vi "Automatic Teller Machine (ATM).vi"() -> ()   [LabVIEW 2015]
uses:
  Controls/State.ctl
  Controls/AccessModeFGV.ctl
panel:
  in  "Enter":bool
  in  "User Input":string
  in  "Right Buttons":T1
  out "Right Menu":T2
  in  "Left Buttons":T1
  out "Left Menu":T2
  in  "Card Simulator":bool
  out "ATM Messages":string
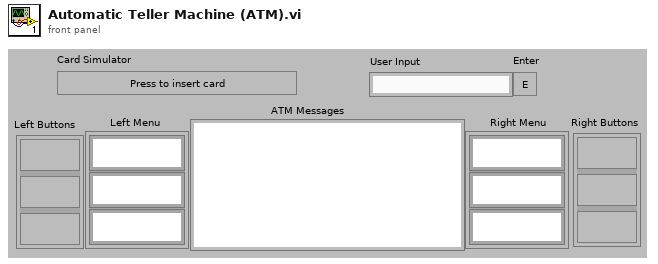
[diagram p1: front panel]
types:
  T1 = cluster{"Func Button":bool, "Func Button 2":bool, "Func Button 3":bool}
  T2 = cluster{"RFS String":string, "RFS String 2":string, "RFS String 3":string}
  T3 = typedef "AccessModeFGV.ctl" = enum16{"SearchUser", "Deposite", "Withdraw", "Fast Cash $50", "Balance Inquiry"}
  T4 = typedef "State.ctl" = enum16{"Init", "Start", "Work", "Stop"}
  T5 = enum8{"Enabled", "Disabled", "Disabled and Grayed Out"}
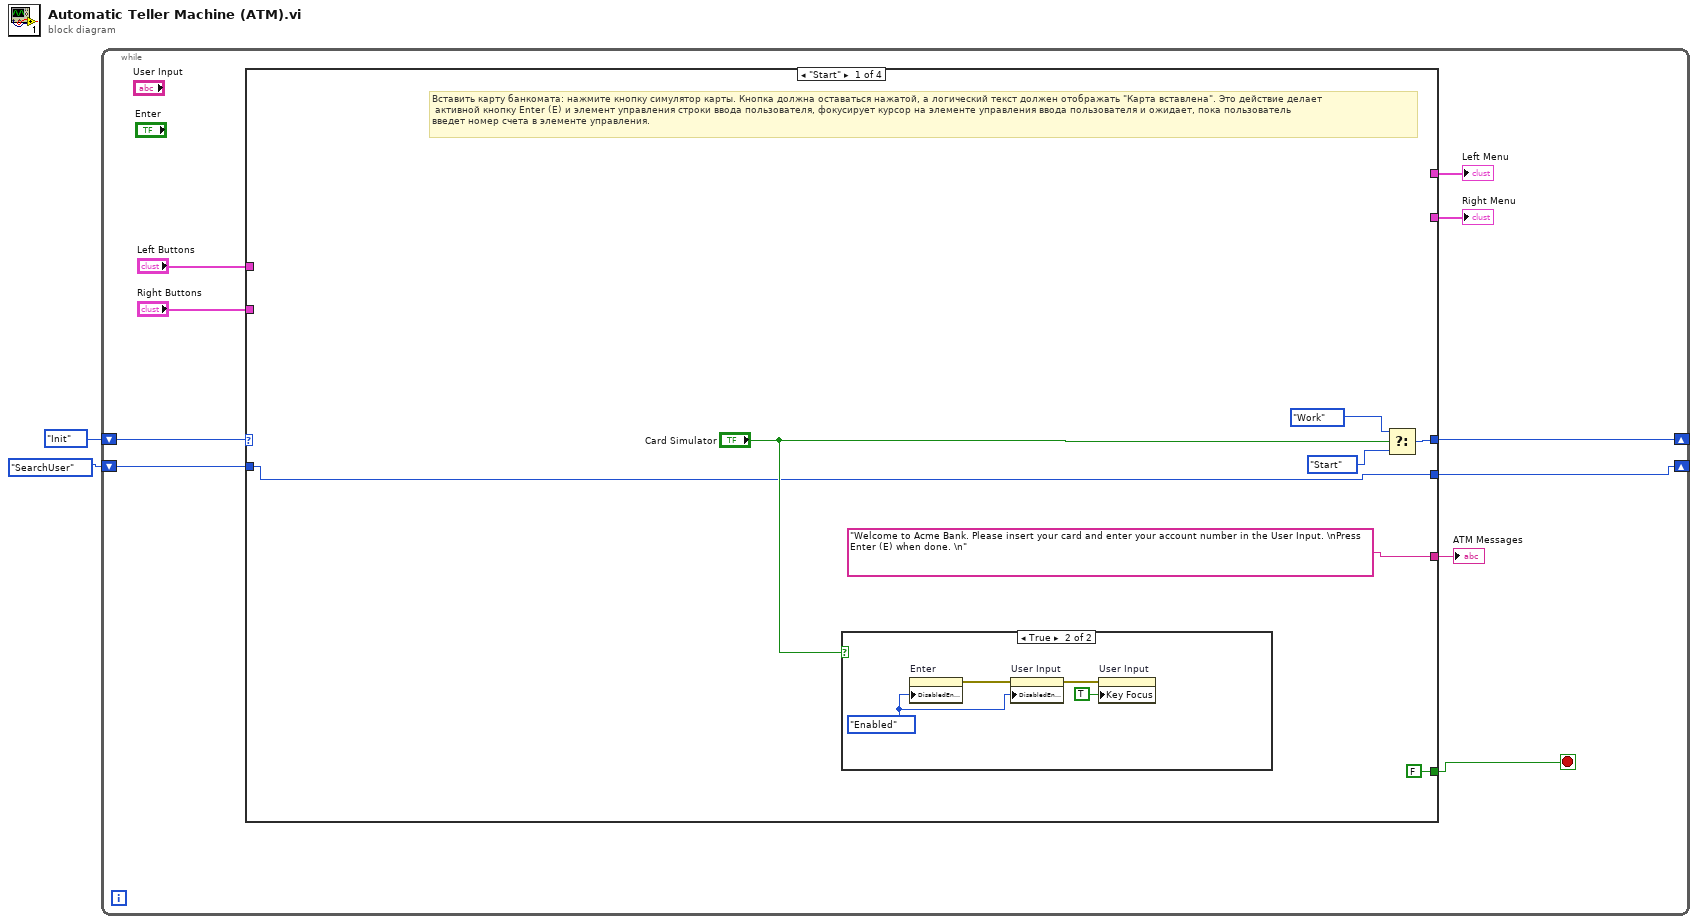
[diagram p0: block diagram]
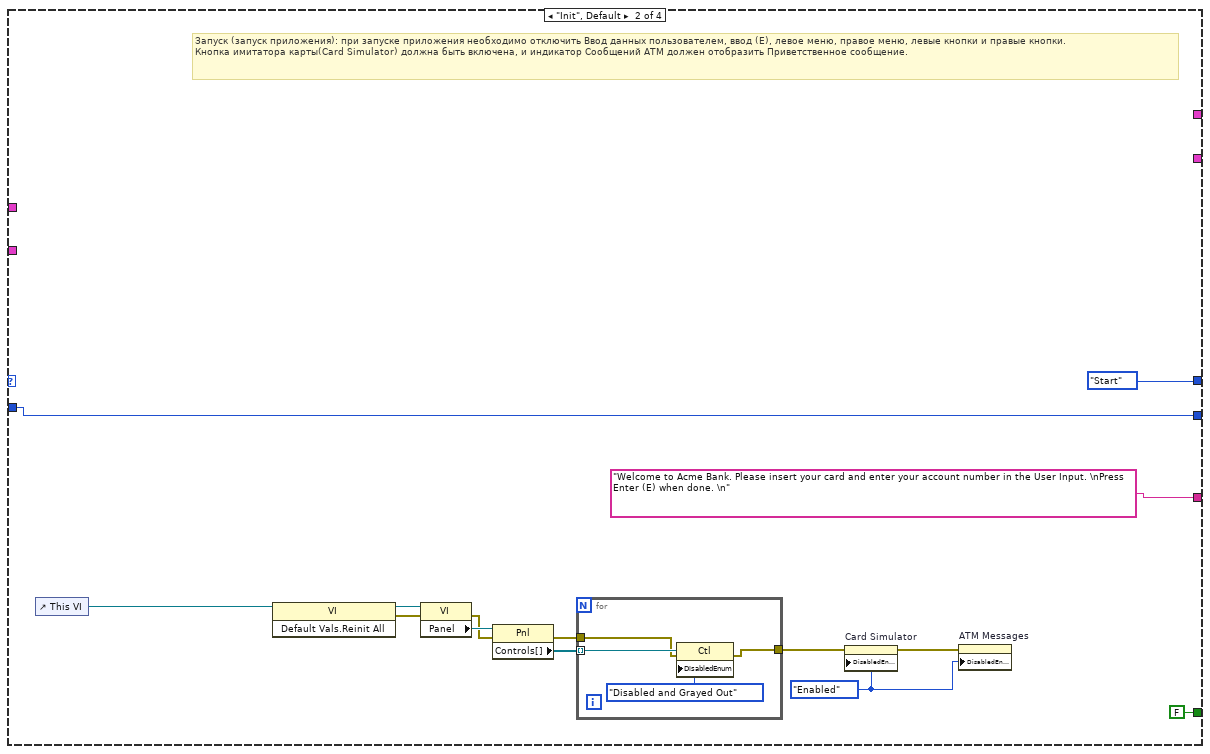
[diagram p3: hidden frame]
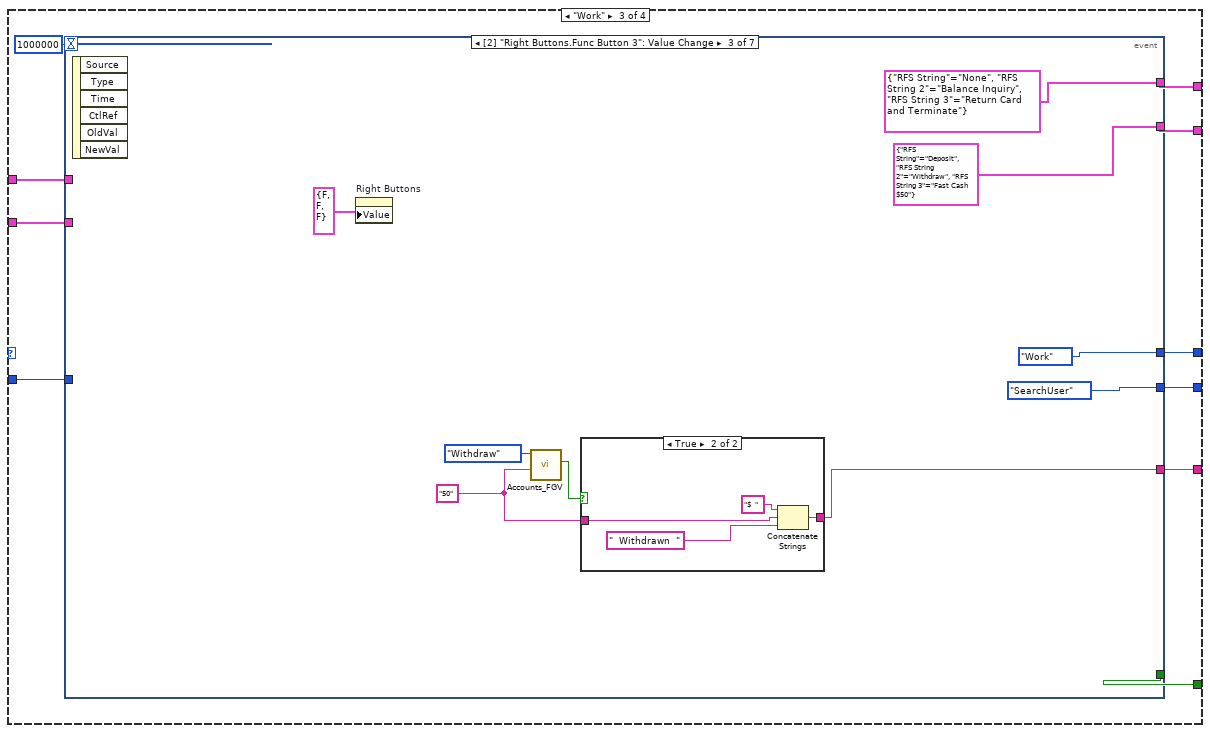
[diagram p4: hidden frame]
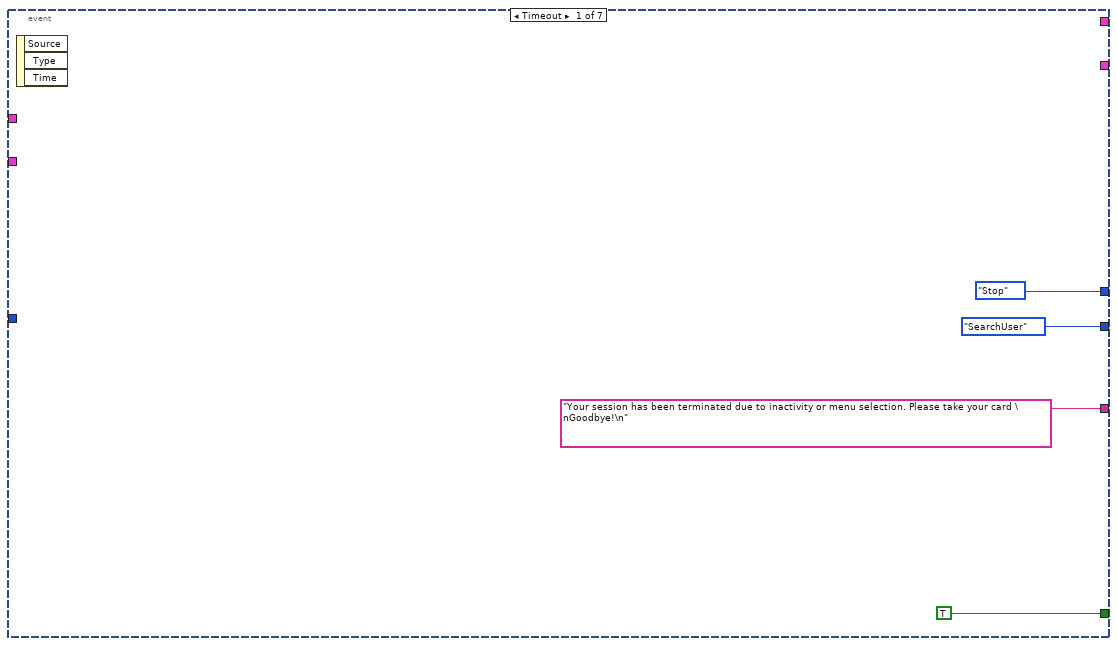
[diagram p5: hidden frame]
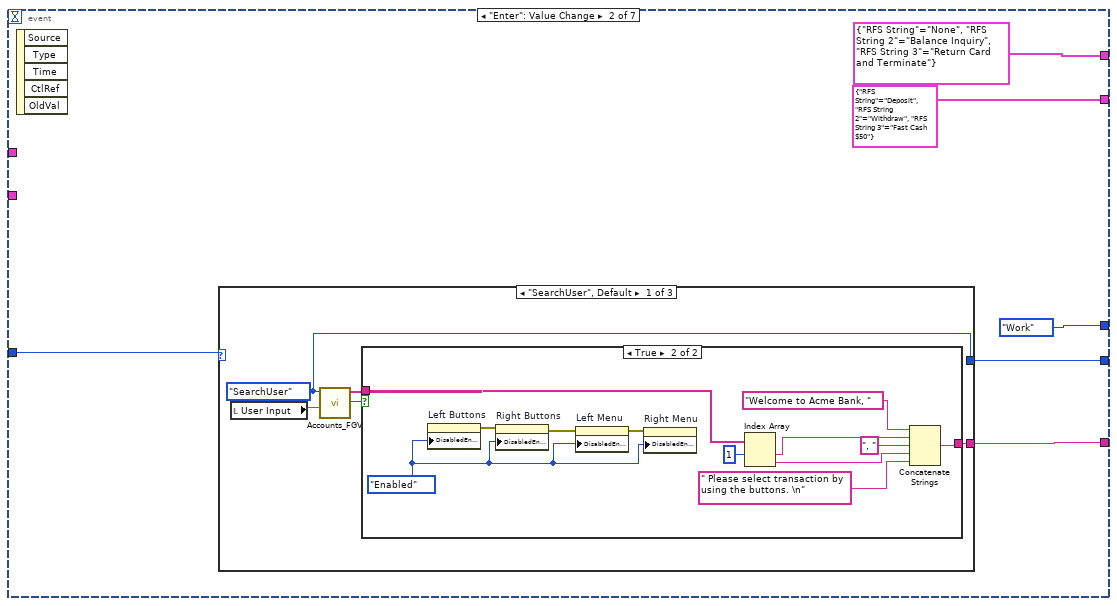
[diagram p6: hidden frame]
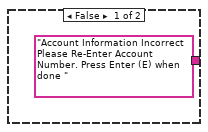
[diagram p7: hidden frame]
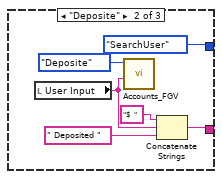
[diagram p8: hidden frame]
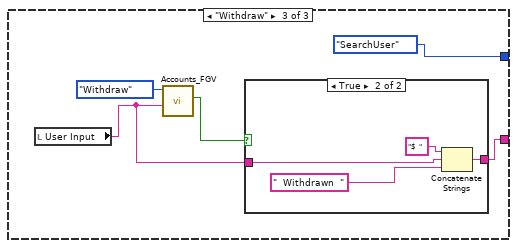
[diagram p9: hidden frame]
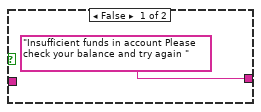
[diagram p10: hidden frame]
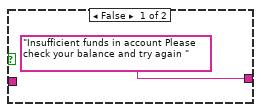
[diagram p11: hidden frame]
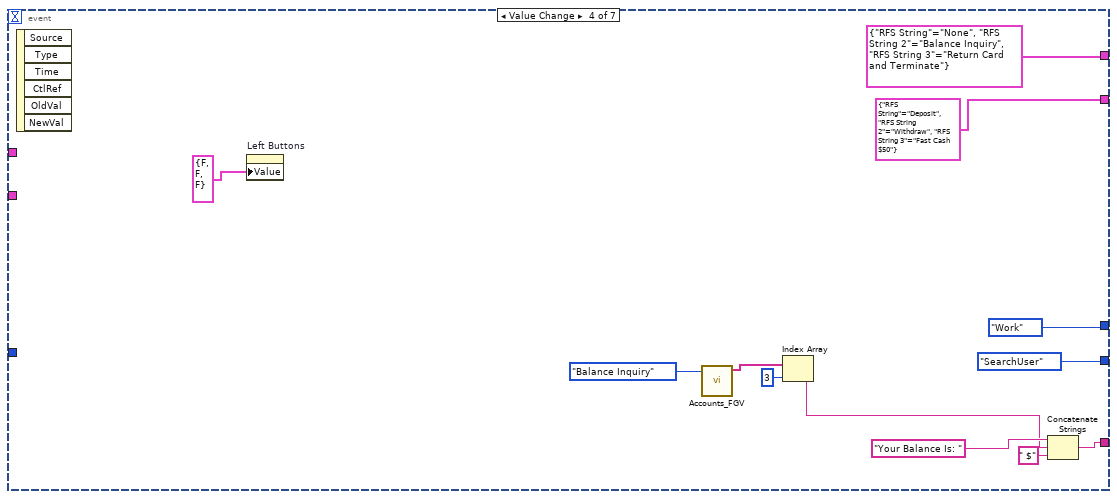
[diagram p12: hidden frame]
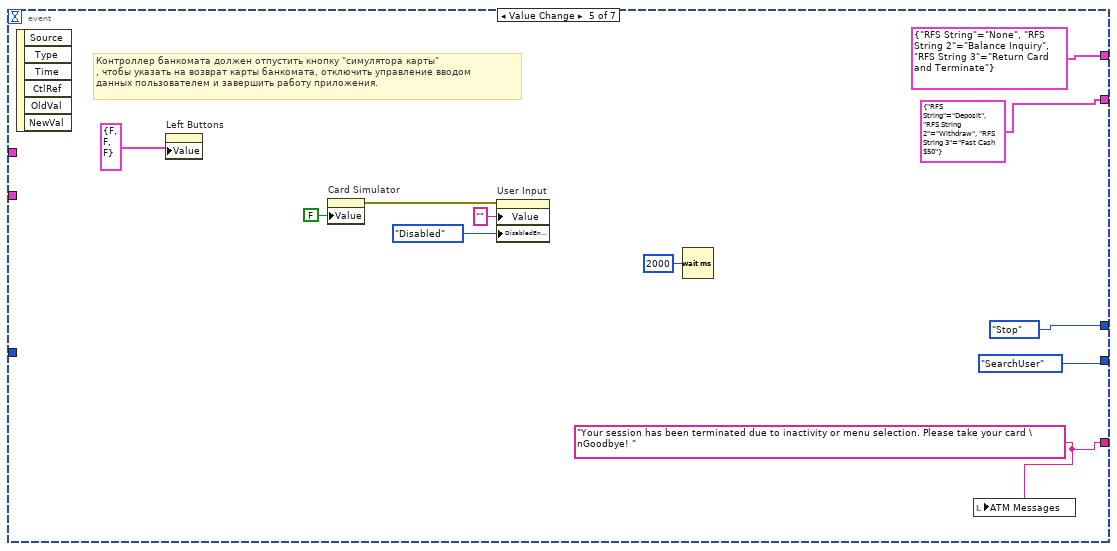
[diagram p13: hidden frame]
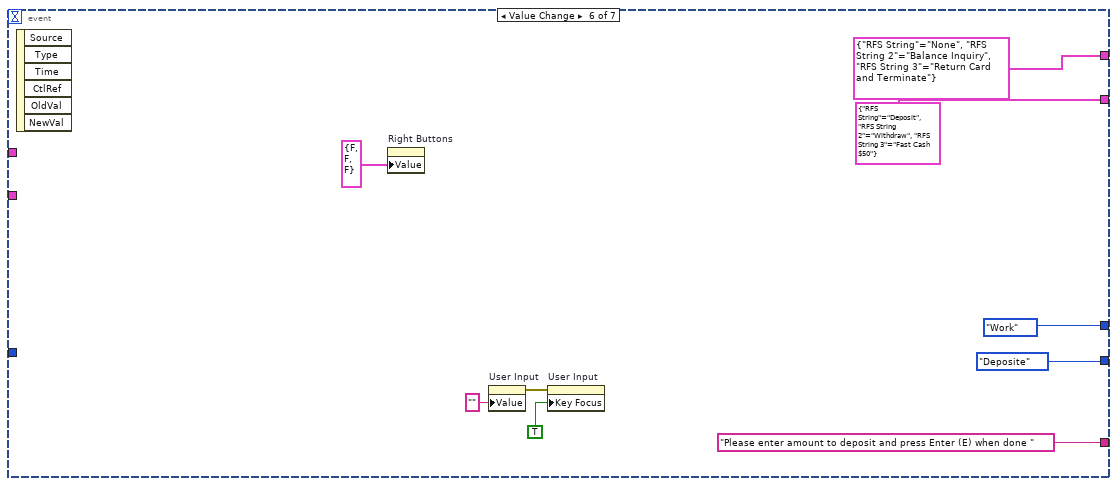
[diagram p14: hidden frame]
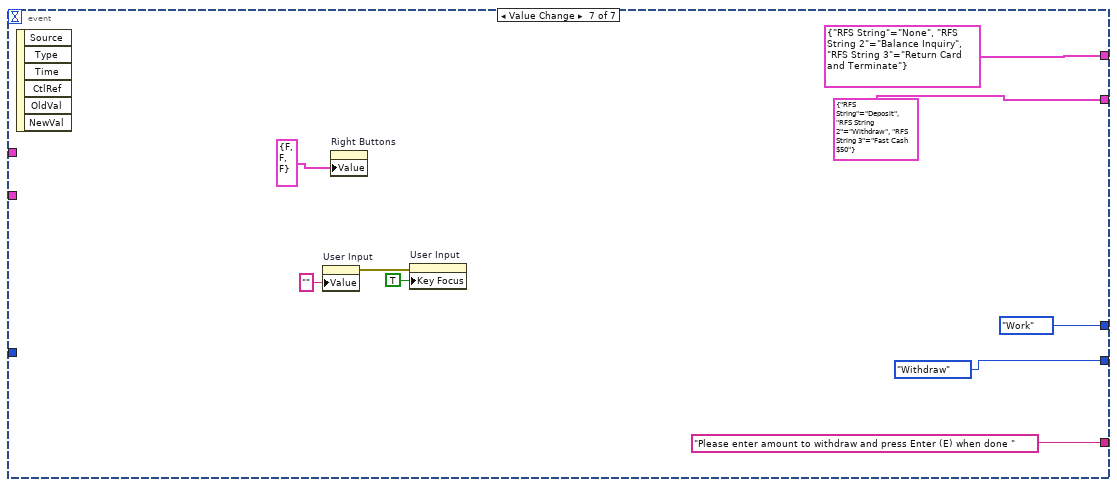
[diagram p15: hidden frame]
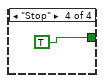
[diagram p16: hidden frame]
diagram:
  n1 = while {
    shift-right: [w11] -> _
    shift-left: State."Init" ("Mode") -> [w12]
    shift-right: [w4] -> _
    shift-left: AccessModeFGV."SearchUser" ("Access mode") -> [w5]
    stop <- w3 stop-if-true
    n2 = case shown="\"Start\"" w12 {
      tunnel: [w17 State."Start" ("Mode") w48 _] -> w11
      tunnel: ["Welcome to Acme Bank. Please insert your card and enter your account number in the User Input. \nPress Enter (E) when done. \n" "Welcome to Acme Bank. Please insert your card and enter your account number in the User Input. \nPress Enter (E) when done. \n" w49 _] -> w10
      tunnel: [FALSE FALSE w50 TRUE] -> w3
      tunnel: "Left Buttons" -> [_ _ w47 _]
      tunnel: "Right Buttons" -> [_ _ w46 _]
      tunnel: [_ _ w45 _] -> w7
      tunnel: [_ _ w44 _] -> w6
      tunnel: w5 -> [w13 w24 w43 _]
      tunnel: [w13 w24 w42 _] -> w4
      frame "Start" {
        # "Вставить карту банкомата: нажмите кнопку симулятор карты. Кнопка должна оставаться нажатой, а логический текст должен отображать \"Карта вставлена\". Это действие делает\n активной кнопку Enter (E) и элемент управления строки ввода пользователя, фокусирует курсор на элементе управления ввода пользователя и ожидает, пока пользователь \nвведет номер счета в элементе управления."
        n3 = case shown="True" "Card Simulator" {
          frame False {
          }
          frame True {
            w22 = T5."Enabled" ("Disabled")
            n4 = property on="Enter" class="Bool"("DisabledEnum"=w22) -> (error out=w23:errorcluster)  [unwired: 2 in, 1 out]
            n5 = property on="User Input" class="Str"(error in=w23, "DisabledEnum"=w22) -> (error out=w21:errorcluster)  [unwired: 1 in, 1 out]
            n6 = property on="User Input" class="Str"(error in=w21, "Key Focus"=TRUE) -> ()  [unwired: 1 in, 2 out]
          }
        }
        n7 = Select(t=State."Work" ("Mode"), s="Card Simulator", f=State."Start" ("Mode")) -> (s? t:f=w17:T4)
      }
      frame "Init", Default {
        w33 = T5."Enabled" ("Disabled")
        # "Запуск (запуск приложения): при запуске приложения необходимо отключить Ввод данных пользователем, ввод (E), левое меню, правое меню, левые кнопки и правые кнопки.\nКнопка имитатора карты(Card Simulator) должна быть включена, и индикатор Сообщений ATM должен отобразить Приветственное сообщение."
        n8 = control-ref of="This VI"() -> (w37:refnum<vi>)
        n9 = invoke class="VI" method="Default Vals.Reinit All"(reference=w37) -> (reference out=w36:refnum<vi>, error out=w32:errorcluster)  [unwired: 2 in, 1 out]
        n10 = property class="VI"(reference=w36, error in=w32) -> (error out=w31:errorcluster, "Panel"=w35:refnum<vi>)  [unwired: 1 out]
        n11 = property class="Pnl"(reference=w35, error in=w31) -> (error out=w30:errorcluster, "Controls[]"=w34:refnum<vi>[])  [unwired: 1 out]
        n12 = for {
          tunnel: w34 -> [w41] mode=indexing
          tunnel: w30 -> [w39]
          tunnel: [w38] -> w29
          n13 = property class="Ctl"(reference=w41, error in=w39, "DisabledEnum"=T5."Disabled and Grayed Out" ("Disabled")) -> (error out=w38:errorcluster)  [unwired: 1 out]
        }
        n14 = property on="Card Simulator" class="Bool (strict)"(error in=w29, "DisabledEnum"=w33) -> (error out=w28:errorcluster)  [unwired: 1 in, 1 out]
        n15 = property on="ATM Messages" class="Str"(error in=w28, "DisabledEnum"=w33) -> ()  [unwired: 1 in, 2 out]
      }
      frame "Work" {
        n16 = event shown="[2] \"Right Buttons.Func Button 3\": Value Change" {
          selector: _ -> [_ _ _ _ _ _ _]
          dyn-events: _ -> [_ _ _ _ _ _ _]
          timeout: 1000000 -> [_ _ _ _ _ _ _]
          tunnel: [TRUE _ _ _ _ _ _] -> w50
          tunnel: ["Your session has been terminated due to inactivity or menu selection. Please take your card \nGoodbye!\n" w61 w97 w110 w122 "Please enter amount to deposit and press Enter (E) when done " "Please enter amount to withdraw and press Enter (E) when done "] -> w49
          tunnel: [State."Stop" ("Mode") State."Work" ("Mode") State."Work" ("Mode") State."Work" ("Mode") State."Stop" ("Mode") State."Work" ("Mode") State."Work" ("Mode")] -> w48
          tunnel: w47 -> [_ _ _ _ _ _ _]
          tunnel: w46 -> [_ _ _ _ _ _ _]
          tunnel: [_ T2 {"RFS String"="None", "RFS String 2"="Balance Inquiry", "RFS String 3"="Return Card and Terminate"} ("Left Menu") T2 {"RFS String"="None", "RFS String 2"="Balance Inquiry", "RFS String 3"="Return Card and Terminate"} ("Left Menu") T2 {"RFS String"="None", "RFS String 2"="Balance Inquiry", "RFS String 3"="Return Card and Terminate"} ("Left Menu") T2 {"RFS String"="None", "RFS String 2"="Balance Inquiry", "RFS String 3"="Return Card and Terminate"} ("Left Menu") T2 {"RFS String"="None", "RFS String 2"="Balance Inquiry", "RFS String 3"="Return Card and Terminate"} ("Left Menu") T2 {"RFS String"="None", "RFS String 2"="Balance Inquiry", "RFS String 3"="Return Card and Terminate"} ("Left Menu")] -> w45
          tunnel: [_ T2 {"RFS String"="Deposit", "RFS String 2"="Withdraw", "RFS String 3"="Fast Cash $50"} ("Left Menu") T2 {"RFS String"="Deposit", "RFS String 2"="Withdraw", "RFS String 3"="Fast Cash $50"} ("Left Menu") T2 {"RFS String"="Deposit", "RFS String 2"="Withdraw", "RFS String 3"="Fast Cash $50"} ("Left Menu") T2 {"RFS String"="Deposit", "RFS String 2"="Withdraw", "RFS String 3"="Fast Cash $50"} ("Left Menu") T2 {"RFS String"="Deposit", "RFS String 2"="Withdraw", "RFS String 3"="Fast Cash $50"} ("Left Menu") T2 {"RFS String"="Deposit", "RFS String 2"="Withdraw", "RFS String 3"="Fast Cash $50"} ("Left Menu")] -> w44
          tunnel: w43 -> [_ w57 _ _ _ _ _]
          tunnel: [AccessModeFGV."SearchUser" ("Access mode") w56 AccessModeFGV."SearchUser" ("Access mode") AccessModeFGV."SearchUser" ("Access mode") AccessModeFGV."SearchUser" ("Access mode") AccessModeFGV."Deposite" ("Access mode") AccessModeFGV."Withdraw" ("Access mode")] -> w42
          event Timeout {
            n17 = event-data() -> ()  [unwired: 1 in, 3 out]
          }
          event "Enter": Value Change {
            n18 = event-data() -> ()  [unwired: 1 in, 5 out]
            n19 = case shown="\"SearchUser\", Default" w57 {
              tunnel: [w64 w81 w87] -> w61
              tunnel: [w62 AccessModeFGV."SearchUser" ("Access mode") AccessModeFGV."SearchUser" ("Access mode")] -> w56
              frame "SearchUser", Default {
                w62 = AccessModeFGV."SearchUser" ("Access mode")
                n20 = local read "User Input"() -> (w66:string)
                n21 = call "Accounts_FGV.vi"("User Input"=w66, "Access mode"=w62) -> ("Find"=w65:bool, "User Info"=w63:string[])  [unwired: 8 in]
                n22 = case shown="True" w65 {
                  tunnel: ["Account Information Incorrect Please Re-Enter Account Number. Press Enter (E) when done " w72] -> w64
                  tunnel: w63 -> [_ w78]
                  frame False {
                  }
                  frame True {
                    w68 = T5."Enabled" ("Disabled")
                    n23 = property on="Left Buttons" class="Clust"("DisabledEnum"=w68) -> (error out=w71:errorcluster)  [unwired: 2 in, 1 out]
                    n24 = property on="Right Buttons" class="Clust"(error in=w71, "DisabledEnum"=w68) -> (error out=w69:errorcluster)  [unwired: 1 in, 1 out]
                    n25 = property on="Left Menu" class="Clust (strict)"(error in=w69, "DisabledEnum"=w68) -> (error out=w70:errorcluster)  [unwired: 1 in, 1 out]
                    n26 = property on="Right Menu" class="Clust (strict)"(error in=w70, "DisabledEnum"=w68) -> ()  [unwired: 1 in, 2 out]
                    n27 = Index Array(array=w78, index #1=1 ("index")) -> (element #1=w76:string, element #2=w74:string)  [unwired: 1 in]
                    n28 = Concatenate Strings("Welcome to Acme Bank, ", w76, ", " ("string"), w74, " Please select transaction by using the buttons. \n") -> (w72:string)
                  }
                }
              }
              frame "Deposite" {
                n29 = local read "User Input"() -> (w82:string)
                n30 = call "Accounts_FGV.vi"("User Input"=w82, "Access mode"=AccessModeFGV."Deposite") -> ()  [unwired: 8 in, 2 out]
                n31 = Concatenate Strings("$  ", w82, " Deposited ") -> (w81:string)
              }
              frame "Withdraw" {
                n32 = local read "User Input"() -> (w88:string)
                n33 = call "Accounts_FGV.vi"("User Input"=w88, "Access mode"=AccessModeFGV."Withdraw") -> ("Find"=w86:bool)  [unwired: 8 in, 1 out]
                n34 = case shown="True" w86 {
                  tunnel: w88 -> [_ w93]
                  tunnel: ["Insufficient funds in account Please check your balance and try again " w92] -> w87
                  frame False {
                  }
                  frame True {
                    n35 = Concatenate Strings("$  ", w93, "  Withdrawn  ") -> (w92:string)
                  }
                }
              }
            }
          }
          event "Right Buttons.Func Button 3": Value Change {
            w98 = "50" ("User Input")
            n36 = event-data() -> ()  [unwired: 1 in, 6 out]
            n37 = property on="Right Buttons" class="Clust"("Value"=T1 {"Func Button"=FALSE, "Func Button 2"=FALSE, "Func Button 3"=FALSE} ("Left Buttons")) -> ()  [unwired: 2 in, 2 out]
            n38 = call "Accounts_FGV.vi"("User Input"=w98, "Access mode"=AccessModeFGV."Withdraw") -> ("Find"=w99:bool)  [unwired: 8 in, 1 out]
            n39 = case shown="True" w99 {
              tunnel: w98 -> [_ w107]
              tunnel: ["Insufficient funds in account Please check your balance and try again " w106] -> w97
              frame False {
              }
              frame True {
                n40 = Concatenate Strings("$  ", w107, "  Withdrawn  ") -> (w106:string)
              }
            }
          }
          event "Left Buttons.Func Button 2": Value Change {
            n41 = event-data() -> ()  [unwired: 1 in, 6 out]
            n42 = property on="Left Buttons" class="Clust"("Value"=T1 {"Func Button"=FALSE, "Func Button 2"=FALSE, "Func Button 3"=FALSE} ("Left Buttons")) -> ()  [unwired: 2 in, 2 out]
            n43 = call "Accounts_FGV.vi"("Access mode"=AccessModeFGV."Balance Inquiry") -> ("User Info"=w115:string[])  [unwired: 9 in, 1 out]
            n44 = Index Array(array=w115, index=3) -> (element=w112:string)
            n45 = Concatenate Strings("Your Balance Is: ", w112, " $" ("string")) -> (w110:string)
          }
          event "Left Buttons.Func Button 3": Value Change {
            w122 = "Your session has been terminated due to inactivity or menu selection. Please take your card \nGoodbye! "
            # "Контроллер банкомата должен отпустить кнопку \"симулятора карты\"\n, чтобы указать на возврат карты банкомата, отключить управление вводом \nданных пользователем и завершить работу приложения."
            n46 = event-data() -> ()  [unwired: 1 in, 6 out]
            n47 = property on="Left Buttons" class="Clust"("Value"=T1 {"Func Button"=FALSE, "Func Button 2"=FALSE, "Func Button 3"=FALSE} ("Left Buttons")) -> ()  [unwired: 2 in, 2 out]
            n48 = property on="Card Simulator" class="Bool (strict)"("Value"=FALSE ("Card Simulator")) -> (error out=w126:errorcluster)  [unwired: 2 in, 1 out]
            n49 = property on="User Input" class="Str"(error in=w126, "Value"="" ("User Input"), "DisabledEnum"=T5."Disabled" ("Disabled")) -> ()  [unwired: 1 in, 2 out]
            n50 = Wait (ms)(milliseconds to wait=u32 2000) -> ()  [unwired: 1 out]
            n51 = local write "ATM Messages"(w122) -> ()
          }
          event "Right Buttons.Func Button": Value Change {
            n52 = event-data() -> ()  [unwired: 1 in, 6 out]
            n53 = property on="Right Buttons" class="Clust"("Value"=T1 {"Func Button"=FALSE, "Func Button 2"=FALSE, "Func Button 3"=FALSE} ("Left Buttons")) -> ()  [unwired: 2 in, 2 out]
            n54 = property on="User Input" class="Str"("Value"="" ("User Input")) -> (error out=w136:errorcluster)  [unwired: 2 in, 1 out]
            n55 = property on="User Input" class="Str"(error in=w136, "Key Focus"=TRUE) -> ()  [unwired: 1 in, 2 out]
          }
          event "Right Buttons.Func Button 2": Value Change {
            n56 = event-data() -> ()  [unwired: 1 in, 6 out]
            n57 = property on="User Input" class="Str"("Value"="" ("User Input")) -> (error out=w146:errorcluster)  [unwired: 2 in, 1 out]
            n58 = property on="Right Buttons" class="Clust"("Value"=T1 {"Func Button"=FALSE, "Func Button 2"=FALSE, "Func Button 3"=FALSE} ("Left Buttons")) -> ()  [unwired: 2 in, 2 out]
            n59 = property on="User Input" class="Str"(error in=w146, "Key Focus"=TRUE) -> ()  [unwired: 1 in, 2 out]
          }
        }
      }
      frame "Stop" {
      }
    }
    "ATM Messages" <- w10
    "Left Menu" <- w7
    "Right Menu" <- w6
  }
